vi "剖面多参数上传.vi"(11 "错误输入（无错误）":errorcluster) -> (15 "error out":errorcluster)   [LabVIEW 2016, in "数据传输系统-02.lvlib"]
uses:
  <vilib>/Utility/config.llb/Write Key (String).vi
  <vilib>/Utility/config.llb/Read Key (String).vi
  <vilib>/Utility/config.llb/NI_LVConfig.lvlib
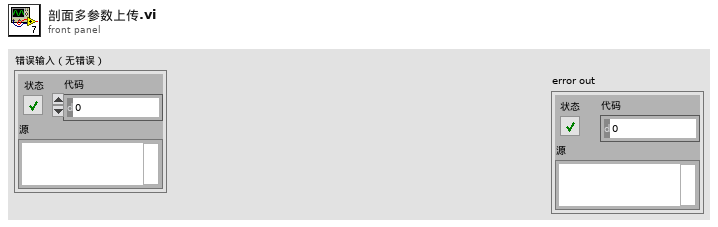
[diagram p1: front panel]
types:
  T1 = cluster{"setini":string, "sysini":string, "hechaini":string, "actualwrite":string, "actualread":string, "datasent":string, "反控命令信息队列":string, "反控与仪器交互":string}
  T2 = typedef "NI_LVConfig.lvlib/Config Data RefNum.ctl" = refnum<k1>
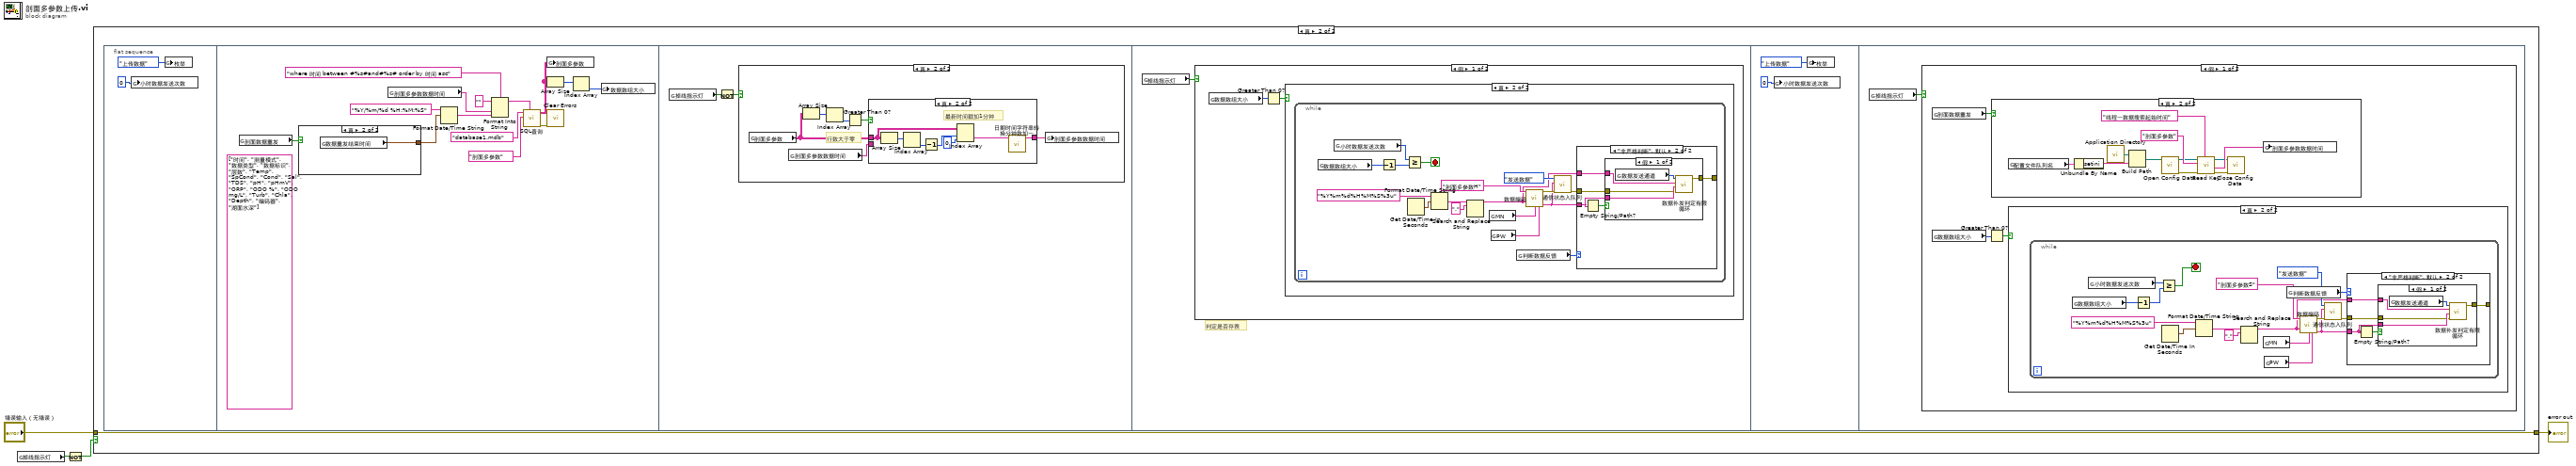
[diagram p0: block diagram]
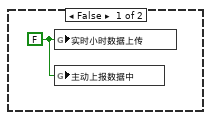
[diagram p2: hidden frame]
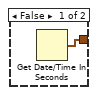
[diagram p3: hidden frame]
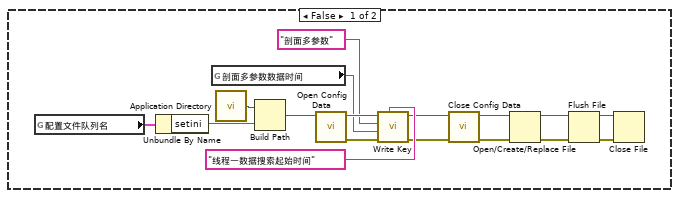
[diagram p10: hidden frame]
diagram:
  n1 = global read "全局 数据发送重叠.vi" "掉线指示灯"() -> (w4:bool)
  n2 = Not(x=w4) -> (.not. x?=w1:bool)
  n3 = case shown="真" w1 {
    tunnel: [_ w6] -> w3
    tunnel: "错误输入（无错误）" -> [_ w6]
    frame False {
      w5 = FALSE ("小时数据上传")
      n4 = global write "全局1.vi" "实时小时数据上传"(w5) -> ()
      n5 = global write "全局 数据发送重叠.vi" "主动上报数据中"(w5) -> ()
    }
    frame True {
      n6 = flat-sequence {
        frame #0 {
          n7 = global write "全局 小时数据发送次数.vi" "小时数据发送次数"(0 ("小时数据发送次数")) -> ()
          n8 = global write "全局1.vi" "枚举"(enum16{"返回请求应答", "上传数据", "返回执行结果"}."上传数据" ("枚举")) -> ()
        }
        frame #1 {
          (unwired) string[] ["时间", "测量模式", "数据类型", "数据标识", "层数", "Temp", "SpCond", "Cond", "Sal", "TDS", "pH", "pHmV", "ORP", "ODO %", "ODO mg/L", "Turb", "Chla", "Depth", "编码器", "湖面水深"] ("columns 2")
          n9 = global read "断电保存全局.vi" "剖面数据重发"() -> (w10:bool)
          n10 = case shown="真" w10 {
            tunnel: [w23 w24] -> w9
            frame False {
              n11 = Get Date/Time In Seconds() -> (seconds since 1Jan1904=w23:timestamp)
            }
            frame True {
              n12 = global read "断电保存全局.vi" "数据重发结束时间"() -> (w24:timestamp)
            }
          }
          n13 = global read "全局 水样时间.vi" "剖面多参数数据时间"() -> (w17:string)
          n14 = Format Date/Time String(time format string (%c)="%Y/%m/%d %H:%M:%S" ("时间格式字符串(%c)"), seconds (now)=w9) -> (date/time string=w16:string)  [unwired: 1 in]
          n15 = Format Into String(format string="where 时间 between #%s#and#%s# order by 时间 asc" ("condition"), initial string="" ("初始字符串"), w17, w16) -> (resulting string=w15:string)  [unwired: 1 in, 1 out]
          n16 = call "SQL查询.vi"("condition"=w15, "table输入"="剖面多参数", "database"="database1.mdb") -> ("error out"=w11:errorcluster, "data"=w14:string[][])  [unwired: 5 in, 2 out]
          n17 = global write "全局 所有参数.vi" "剖面多参数"(w14) -> ()
          n18 = Array Size(array=w14) -> (size(s)=w13:i32[])
          n19 = call <vilib>:"Clear Errors.vi"("error in (no error)"=w11) -> ()  [unwired: 5 in, 2 out]
          n20 = Index Array(array=w13) -> (element=w12:i32)  [unwired: 1 in]
          n21 = global write "全局 数据数组大小.vi" "数据数组大小"(w12) -> ()
        }
        frame #2 {
          n22 = global read "全局 数据发送重叠.vi" "掉线指示灯"() -> (w26:bool)
          n23 = Not(x=w26) -> (.not. x?=w25:bool)
          n24 = case shown="真" w25 {
            frame False {
            }
            frame True {
              # "行数大于零"
              n25 = global read "全局 所有参数.vi" "剖面多参数"() -> (w31:string[][])
              n26 = global read "全局 水样时间.vi" "剖面多参数数据时间"() -> (w32:string)
              n27 = Array Size(array=w31) -> (size(s)=w28:i32[])
              n28 = Index Array(array=w28) -> (element=w29:i32)  [unwired: 1 in]
              n29 = Greater Than 0?(x=w29) -> (x > 0?=w30:bool)
              n30 = case shown="真" w30 {
                tunnel: w31 -> [_ w37]
                tunnel: [w33 w34] -> w27
                tunnel: w32 -> [w33 _]
                frame False {
                }
                frame True {
                  # "最新时间戳加1分钟"
                  n31 = Array Size(array=w37) -> (size(s)=w39:i32[])
                  n32 = Index Array(array=w39) -> (element=w38:i32)  [unwired: 1 in]
                  n33 = Decrement(x=w38) -> (x-1=w36:i32)
                  n34 = Index Array(array=w37, index (row)=w36, index (col)=0 ("禁用的索引 (列)")) -> (element=w40:string)
                  n35 = call "日期时间字符串转换分钟数加一.vi"("data[0]"=w40) -> ("日期/时间字符串"=w34:string)  [unwired: 10 in]
                }
              }
              n36 = global write "全局 水样时间.vi" "剖面多参数数据时间"(w27) -> ()
            }
          }
        }
        frame #3 {
          # "判定是否存表"
          n37 = global read "全局 数据发送重叠.vi" "掉线指示灯"() -> (w41:bool)
          n38 = case shown="假" w41 {
            frame False {
              n39 = global read "全局 数据数组大小.vi" "数据数组大小"() -> (w42:i32)
              n40 = Greater Than 0?(x=w42) -> (x > 0?=w43:bool)
              n41 = case shown="真" w43 {
                frame False {
                }
                frame True {
                  n42 = while {
                    stop <- w49 stop-if-true
                    n43 = global read "全局 数据数组大小.vi" "数据数组大小"() -> (w51:i32)
                    n44 = global read "全局 小时数据发送次数.vi" "小时数据发送次数"() -> (w52:i32)
                    n45 = Decrement(x=w51) -> (x-1=w50:i32)
                    n46 = Greater Or Equal?(x=w52, y=w50) -> (x >= y?=w49:bool)
                    n47 = Get Date/Time In Seconds() -> (seconds since 1Jan1904=w58:timestamp)
                    n48 = Format Date/Time String(time format string (%c)="%Y%m%d%H%M%S%3u" ("时间格式字符串(%c)"), seconds (now)=w58) -> (date/time string=w57:string)  [unwired: 1 in]
                    n49 = Search and Replace String(input string=w57, search string="." ("搜索字符串")) -> (result string=w46:string)  [unwired: 6 in, 3 out]
                    n50 = global read "断电保存全局.vi" "MN"() -> (w55:string)
                    n51 = global read "断电保存全局.vi" "PW"() -> (w54:string)
                    n52 = global read "断电保存全局.vi" "判断数据反馈"() -> (w47:enum16{"非严格判断", "严格判断", "不判断"})
                    n53 = call "数据编码.vi"("table输入"="剖面多参数H" ("新元素/子数组"), "QN"=w46, "MN"=w55, "PW"=w54) -> ("错误常量"=w53:errorcluster, "通讯包字符串"=w45:string)  [unwired: 10 in]
                    n54 = call "通信状态入队列.vi"("错误输入（无错误）"=w53, "发送报文"=w45, "枚举"=enum16{"打开连接", "发送数据", "读取数据", "数据处理", "关闭连接"}."发送数据") -> ("错误输出"=w44:errorcluster)  [unwired: 8 in]
                    n55 = case shown="\"非严格判断\", 默认" w47 {
                      tunnel: [_ w65] -> _
                      tunnel: w45 -> [_ w64]
                      tunnel: w46 -> [_ w63]
                      tunnel: w44 -> [_ w61]
                      frame "不判断" {
                      }
                      frame "非严格判断", Default {
                        n56 = Empty String/Path?(string/path=w64) -> (empty?=w62:bool)
                        n57 = case shown="假" w62 {
                          tunnel: [w70 _] -> w65
                          tunnel: w64 -> [w69 _]
                          tunnel: w63 -> [w67 _]
                          tunnel: w61 -> [w66 _]
                          frame False {
                            n58 = global read "断电保存全局.vi" "数据发送通道"() -> (w68:enum16{"TCP", "VISA"})
                            n59 = call "数据补发判定有限循环.vi"("错误输入（无错误）"=w66, "数据输入"=w69, "QN"=w67, "数据发送通道"=w68) -> ("error out"=w70:errorcluster)  [unwired: 7 in]
                          }
                          frame True {
                          }
                        }
                      }
                    }
                  }
                }
              }
            }
            frame True {
            }
          }
        }
        frame #4 {
          n60 = global write "全局 小时数据发送次数.vi" "小时数据发送次数"(0 ("小时数据发送次数")) -> ()
          n61 = global write "全局1.vi" "枚举"(enum16{"返回请求应答", "上传数据", "返回执行结果"}."上传数据" ("枚举")) -> ()
        }
        frame #5 {
          n62 = global read "全局 数据发送重叠.vi" "掉线指示灯"() -> (w73:bool)
          n63 = case shown="假" w73 {
            frame False {
              n64 = global read "断电保存全局.vi" "剖面数据重发"() -> (w74:bool)
              n65 = global read "全局 数据数组大小.vi" "数据数组大小"() -> (w76:i32)
              n66 = Greater Than 0?(x=w76) -> (x > 0?=w75:bool)
              n67 = case shown="真" w74 {
                frame False {
                  n68 = global read "全局1.vi" "配置文件队列名"() -> (w77:T1)
                  n69 = Unbundle By Name(w77) -> ("setini"=w78:string)
                  n70 = global read "全局 水样时间.vi" "剖面多参数数据时间"() -> (w79:string)
                  n71 = call <vilib>:"Application Directory.vi"() -> ("Application Directory"=w87:path)
                  n72 = Build Path(base path=w87, name or relative path=w78) -> (appended path=w88:path)
                  n73 = call <vilib>:"Open Config Data.vi"("configuration file path"=w88) -> ("error out"=w90:errorcluster, "refnum"=w89:T2)  [unwired: 8 in, 1 out]
                  n74 = call-poly <vilib>:"Write Key.vi"("section"="线程一数据搜索起始时间", "error in (no error)"=w90, "value"=w79, "key"="剖面多参数", "refnum"=w89) -> ("error out"=w92:errorcluster, "refnum out"=w91:T2)  [unwired: 4 in, 1 out]
                  n75 = call <vilib>:"Close Config Data.vi"("error in (no error)"=w92, "refnum"=w91) -> ("error out"=w80:errorcluster, "file path"=w81:path)  [unwired: 8 in]
                  n76 = Open/Create/Replace File(file path (use dialog)=w81, error in=w80) -> (refnum out=w83:refnum<file>, error out=w82:errorcluster)  [unwired: 4 in, 1 out]
                  n77 = Flush File(refnum=w83, error in=w82) -> (refnum out=w84:refnum<file>, error out=w85:errorcluster)
                  n78 = Close File(refnum=w84, error in=w85) -> ()  [unwired: 2 out]
                }
                frame True {
                  n79 = global read "全局1.vi" "配置文件队列名"() -> (w94:T1)
                  n80 = Unbundle By Name(w94) -> ("setini"=w101:string)
                  n81 = call <vilib>:"Application Directory.vi"() -> ("Application Directory"=w100:path)
                  n82 = Build Path(base path=w100, name or relative path=w101) -> (appended path=w102:path)
                  n83 = call <vilib>:"Open Config Data.vi"("configuration file path"=w102) -> ("error out"=w97:errorcluster, "refnum"=w96:T2)  [unwired: 8 in, 1 out]
                  n84 = call-poly <vilib>:"Read Key.vi"("section"="线程一数据搜索起始时间", "error in (no error)"=w97, "key"="剖面多参数", "refnum"=w96) -> ("error out"=w99:errorcluster, "value"=w104:string, "refnum out"=w98:T2)  [unwired: 4 in, 1 out]
                  n85 = call <vilib>:"Close Config Data.vi"("error in (no error)"=w99, "refnum"=w98) -> ()  [unwired: 8 in, 2 out]
                  n86 = global write "全局 水样时间.vi" "剖面多参数数据时间"(w104) -> ()
                }
              }
              n87 = case shown="真" w75 {
                frame False {
                }
                frame True {
                  n88 = while {
                    stop <- w110 stop-if-true
                    n89 = global read "全局 数据数组大小.vi" "数据数组大小"() -> (w112:i32)
                    n90 = global read "全局 小时数据发送次数.vi" "小时数据发送次数"() -> (w113:i32)
                    n91 = Decrement(x=w112) -> (x-1=w111:i32)
                    n92 = Greater Or Equal?(x=w113, y=w111) -> (x >= y?=w110:bool)
                    n93 = Get Date/Time In Seconds() -> (seconds since 1Jan1904=w119:timestamp)
                    n94 = Format Date/Time String(time format string (%c)="%Y%m%d%H%M%S%3u" ("时间格式字符串(%c)"), seconds (now)=w119) -> (date/time string=w118:string)  [unwired: 1 in]
                    n95 = Search and Replace String(input string=w118, search string="." ("搜索字符串")) -> (result string=w107:string)  [unwired: 6 in, 3 out]
                    n96 = global read "断电保存全局.vi" "MN"() -> (w116:string)
                    n97 = global read "断电保存全局.vi" "PW"() -> (w115:string)
                    n98 = global read "断电保存全局.vi" "判断数据反馈"() -> (w108:enum16{"非严格判断", "严格判断", "不判断"})
                    n99 = call "数据编码.vi"("table输入"="剖面多参数S" ("新元素/子数组"), "QN"=w107, "MN"=w116, "PW"=w115) -> ("错误常量"=w114:errorcluster, "通讯包字符串"=w106:string)  [unwired: 10 in]
                    n100 = call "通信状态入队列.vi"("错误输入（无错误）"=w114, "发送报文"=w106, "枚举"=enum16{"打开连接", "发送数据", "读取数据", "数据处理", "关闭连接"}."发送数据") -> ("错误输出"=w105:errorcluster)  [unwired: 8 in]
                    n101 = case shown="\"非严格判断\", 默认" w108 {
                      tunnel: [_ w126] -> _
                      tunnel: w106 -> [_ w125]
                      tunnel: w107 -> [_ w124]
                      tunnel: w105 -> [_ w122]
                      frame "不判断" {
                      }
                      frame "非严格判断", Default {
                        n102 = Empty String/Path?(string/path=w125) -> (empty?=w123:bool)
                        n103 = case shown="假" w123 {
                          tunnel: [w131 _] -> w126
                          tunnel: w125 -> [w130 _]
                          tunnel: w124 -> [w128 _]
                          tunnel: w122 -> [w127 _]
                          frame False {
                            n104 = global read "断电保存全局.vi" "数据发送通道"() -> (w129:enum16{"TCP", "VISA"})
                            n105 = call "数据补发判定有限循环.vi"("错误输入（无错误）"=w127, "数据输入"=w130, "QN"=w128, "数据发送通道"=w129) -> ("error out"=w131:errorcluster)  [unwired: 7 in]
                          }
                          frame True {
                          }
                        }
                      }
                    }
                  }
                }
              }
            }
            frame True {
            }
          }
        }
      }
    }
  }
  "error out" <- w3
